vi "Emerson 5700 32 Bit Data.vi"(8 "Error In":errorcluster, 10 "Emerson Flow Meter Data Input":T2={"Mass Flow Rate (Scaled Integer)"=65535, "Density (Scaled Integer)"=8, "Temperature (Scaled Integer)"=69, "Volume Flow Rate (Scaled Integer)"=65535, "Totalizer 1 (Scaled Integer)"=65, "Totalizer 2 (Scaled Integer)"=8, "Transmitter Software Rev"=14, "Flow Direction"="Forward", "Mass Flow Units"="lb/min", "Density Units"="lb/US Gal", "Temperature Units"="°F", "Volume Flow Units"="US GPM", "Pressure Units"="PSI", "Mass Total Units"="lbs", "Volume Total Units"="US Gallon", "Inventory 1 (Scaled Integer)"=66, "Inventory 2 (Scaled Integer)"=8, "Mass Flow Rate"=0.0, "Density"=0.0, "Temperature"=0.0, "Volume Flow Rate"=0.0, "Pressure (Scaled Integer)"=40, "Current Value Totalizer 1 (Pounds per draw)"=0.0, "Current Value Totalizer 2 (Gallons per draw)"=0.0, "Current Value Inventory 1 (Pounds Total)"=0.0, "Current Value Inventory 2 (Gallons Total)"=0.0, "Drive Gain"=0.0, "Raw Tube Frequency (Hz)"=0.0, "Dynamic Viscosity (Centipoise)"=0.0, "Kinematic Viscosity (Centistokes)"=0.0, "Hot Gallons (Calculated Gallons)"=0.0, "Hot Flow Rate (Calculated GPM)"=0.0, "Hot Gallons Inventory (Gallons)"=0.0}, 11 "Modbus master in":refnum<class "Modbus Master.lvclass">=refnum) -> (0 "Error Out":errorcluster, 2 "Emerson Flow Meter Data Output":T2, 3 "Modbus master out":refnum<class "Modbus Master.lvclass">)   [LabVIEW 2016]
uses:
  Type Definitions/Emerson 5700 Data.ctl
  <vilib>/NI/Modbus Library/API/Master/Modbus Master.lvclass
  <vilib>/NI/Modbus Library/Transmission Data Unit/IP/IP Data Unit.lvclass
  <vilib>/NI/Modbus Library/Master Function Definition/Master Function Definition.lvclass
  <vilib>/NI/Modbus Library/Network Protocol/Network Master/TCP/TCP Master.lvclass
  Type Definitions/Emerson 5700 Modbus Addresses.ctl
panel:
  in  "CMD 10":T1=291 items=["Kinematic Viscosity-4161"=4161, "Dynamic Viscosity-4159"=4159, "Reset Volume Total (Totalizer 2)-57"=57, "Reset Mass Total (Totalizer 1)-56"=56, "Drive Gain-291"=291, "Raw Tube Frequency (Hz) - 285"=285, "Current Value Inventory 2-265"=265, "Current Value Inventory 1-263"=263, "Current Value Totalizer 2-261"=261, "Current Value Totalizer 1-259"=259, "Volume Flow Rate-253"=253, "Temperature-251"=251, "Density-249"=249, "Mass Flow Rate-247"=247, "Volume Total Unit-46"=46, "Mass Total Unit-45"=45, "Pressure Unit-44"=44, "Volume Flow Unit-42"=42, "Temperature Unit-41"=41, "Density Unit-40"=40, "Mass Flow Units-39"=39, "Flow Direction-17"=17, "Transmitter Software Rev-16"=16, "Inventory 2 (Scaled Integer)-11"=11, "Inventory 1 (Scaled Integer)-10"=10, "Totalizer 2 (Scaled Integer)-9"=9, "Totalizer 1 (Scaled Integer)-8"=8, "Pressure (Scaled Integer) -7"=7, "Volume Flow Rate (Scaled Integer)-5"=5, "Temperature (Scaled Integer)-4"=4, "Density (Scaled Integer)-3"=3, "Mass Flow Rate (Scaled Integer)-2"=2]
  in  "CMD 9":T1=265 items=["Kinematic Viscosity-4161"=4161, "Dynamic Viscosity-4159"=4159, "Reset Volume Total (Totalizer 2)-57"=57, "Reset Mass Total (Totalizer 1)-56"=56, "Drive Gain-291"=291, "Raw Tube Frequency (Hz) - 285"=285, "Current Value Inventory 2-265"=265, "Current Value Inventory 1-263"=263, "Current Value Totalizer 2-261"=261, "Current Value Totalizer 1-259"=259, "Volume Flow Rate-253"=253, "Temperature-251"=251, "Density-249"=249, "Mass Flow Rate-247"=247, "Volume Total Unit-46"=46, "Mass Total Unit-45"=45, "Pressure Unit-44"=44, "Volume Flow Unit-42"=42, "Temperature Unit-41"=41, "Density Unit-40"=40, "Mass Flow Units-39"=39, "Flow Direction-17"=17, "Transmitter Software Rev-16"=16, "Inventory 2 (Scaled Integer)-11"=11, "Inventory 1 (Scaled Integer)-10"=10, "Totalizer 2 (Scaled Integer)-9"=9, "Totalizer 1 (Scaled Integer)-8"=8, "Pressure (Scaled Integer) -7"=7, "Volume Flow Rate (Scaled Integer)-5"=5, "Temperature (Scaled Integer)-4"=4, "Density (Scaled Integer)-3"=3, "Mass Flow Rate (Scaled Integer)-2"=2]
  in  "CMD 8":T1=263 items=["Kinematic Viscosity-4161"=4161, "Dynamic Viscosity-4159"=4159, "Reset Volume Total (Totalizer 2)-57"=57, "Reset Mass Total (Totalizer 1)-56"=56, "Drive Gain-291"=291, "Raw Tube Frequency (Hz) - 285"=285, "Current Value Inventory 2-265"=265, "Current Value Inventory 1-263"=263, "Current Value Totalizer 2-261"=261, "Current Value Totalizer 1-259"=259, "Volume Flow Rate-253"=253, "Temperature-251"=251, "Density-249"=249, "Mass Flow Rate-247"=247, "Volume Total Unit-46"=46, "Mass Total Unit-45"=45, "Pressure Unit-44"=44, "Volume Flow Unit-42"=42, "Temperature Unit-41"=41, "Density Unit-40"=40, "Mass Flow Units-39"=39, "Flow Direction-17"=17, "Transmitter Software Rev-16"=16, "Inventory 2 (Scaled Integer)-11"=11, "Inventory 1 (Scaled Integer)-10"=10, "Totalizer 2 (Scaled Integer)-9"=9, "Totalizer 1 (Scaled Integer)-8"=8, "Pressure (Scaled Integer) -7"=7, "Volume Flow Rate (Scaled Integer)-5"=5, "Temperature (Scaled Integer)-4"=4, "Density (Scaled Integer)-3"=3, "Mass Flow Rate (Scaled Integer)-2"=2]
  in  "CMD 7":T1=261 items=["Kinematic Viscosity-4161"=4161, "Dynamic Viscosity-4159"=4159, "Reset Volume Total (Totalizer 2)-57"=57, "Reset Mass Total (Totalizer 1)-56"=56, "Drive Gain-291"=291, "Raw Tube Frequency (Hz) - 285"=285, "Current Value Inventory 2-265"=265, "Current Value Inventory 1-263"=263, "Current Value Totalizer 2-261"=261, "Current Value Totalizer 1-259"=259, "Volume Flow Rate-253"=253, "Temperature-251"=251, "Density-249"=249, "Mass Flow Rate-247"=247, "Volume Total Unit-46"=46, "Mass Total Unit-45"=45, "Pressure Unit-44"=44, "Volume Flow Unit-42"=42, "Temperature Unit-41"=41, "Density Unit-40"=40, "Mass Flow Units-39"=39, "Flow Direction-17"=17, "Transmitter Software Rev-16"=16, "Inventory 2 (Scaled Integer)-11"=11, "Inventory 1 (Scaled Integer)-10"=10, "Totalizer 2 (Scaled Integer)-9"=9, "Totalizer 1 (Scaled Integer)-8"=8, "Pressure (Scaled Integer) -7"=7, "Volume Flow Rate (Scaled Integer)-5"=5, "Temperature (Scaled Integer)-4"=4, "Density (Scaled Integer)-3"=3, "Mass Flow Rate (Scaled Integer)-2"=2]
  in  "CMD 6":T1=259 items=["Kinematic Viscosity-4161"=4161, "Dynamic Viscosity-4159"=4159, "Reset Volume Total (Totalizer 2)-57"=57, "Reset Mass Total (Totalizer 1)-56"=56, "Drive Gain-291"=291, "Raw Tube Frequency (Hz) - 285"=285, "Current Value Inventory 2-265"=265, "Current Value Inventory 1-263"=263, "Current Value Totalizer 2-261"=261, "Current Value Totalizer 1-259"=259, "Volume Flow Rate-253"=253, "Temperature-251"=251, "Density-249"=249, "Mass Flow Rate-247"=247, "Volume Total Unit-46"=46, "Mass Total Unit-45"=45, "Pressure Unit-44"=44, "Volume Flow Unit-42"=42, "Temperature Unit-41"=41, "Density Unit-40"=40, "Mass Flow Units-39"=39, "Flow Direction-17"=17, "Transmitter Software Rev-16"=16, "Inventory 2 (Scaled Integer)-11"=11, "Inventory 1 (Scaled Integer)-10"=10, "Totalizer 2 (Scaled Integer)-9"=9, "Totalizer 1 (Scaled Integer)-8"=8, "Pressure (Scaled Integer) -7"=7, "Volume Flow Rate (Scaled Integer)-5"=5, "Temperature (Scaled Integer)-4"=4, "Density (Scaled Integer)-3"=3, "Mass Flow Rate (Scaled Integer)-2"=2]
  in  "CMD 5":T1=285 items=["Kinematic Viscosity-4161"=4161, "Dynamic Viscosity-4159"=4159, "Reset Volume Total (Totalizer 2)-57"=57, "Reset Mass Total (Totalizer 1)-56"=56, "Drive Gain-291"=291, "Raw Tube Frequency (Hz) - 285"=285, "Current Value Inventory 2-265"=265, "Current Value Inventory 1-263"=263, "Current Value Totalizer 2-261"=261, "Current Value Totalizer 1-259"=259, "Volume Flow Rate-253"=253, "Temperature-251"=251, "Density-249"=249, "Mass Flow Rate-247"=247, "Volume Total Unit-46"=46, "Mass Total Unit-45"=45, "Pressure Unit-44"=44, "Volume Flow Unit-42"=42, "Temperature Unit-41"=41, "Density Unit-40"=40, "Mass Flow Units-39"=39, "Flow Direction-17"=17, "Transmitter Software Rev-16"=16, "Inventory 2 (Scaled Integer)-11"=11, "Inventory 1 (Scaled Integer)-10"=10, "Totalizer 2 (Scaled Integer)-9"=9, "Totalizer 1 (Scaled Integer)-8"=8, "Pressure (Scaled Integer) -7"=7, "Volume Flow Rate (Scaled Integer)-5"=5, "Temperature (Scaled Integer)-4"=4, "Density (Scaled Integer)-3"=3, "Mass Flow Rate (Scaled Integer)-2"=2]
  in  "CMD 4":T1=253 items=["Kinematic Viscosity-4161"=4161, "Dynamic Viscosity-4159"=4159, "Reset Volume Total (Totalizer 2)-57"=57, "Reset Mass Total (Totalizer 1)-56"=56, "Drive Gain-291"=291, "Raw Tube Frequency (Hz) - 285"=285, "Current Value Inventory 2-265"=265, "Current Value Inventory 1-263"=263, "Current Value Totalizer 2-261"=261, "Current Value Totalizer 1-259"=259, "Volume Flow Rate-253"=253, "Temperature-251"=251, "Density-249"=249, "Mass Flow Rate-247"=247, "Volume Total Unit-46"=46, "Mass Total Unit-45"=45, "Pressure Unit-44"=44, "Volume Flow Unit-42"=42, "Temperature Unit-41"=41, "Density Unit-40"=40, "Mass Flow Units-39"=39, "Flow Direction-17"=17, "Transmitter Software Rev-16"=16, "Inventory 2 (Scaled Integer)-11"=11, "Inventory 1 (Scaled Integer)-10"=10, "Totalizer 2 (Scaled Integer)-9"=9, "Totalizer 1 (Scaled Integer)-8"=8, "Pressure (Scaled Integer) -7"=7, "Volume Flow Rate (Scaled Integer)-5"=5, "Temperature (Scaled Integer)-4"=4, "Density (Scaled Integer)-3"=3, "Mass Flow Rate (Scaled Integer)-2"=2]
  in  "CMD 3":T1=251 items=["Kinematic Viscosity-4161"=4161, "Dynamic Viscosity-4159"=4159, "Reset Volume Total (Totalizer 2)-57"=57, "Reset Mass Total (Totalizer 1)-56"=56, "Drive Gain-291"=291, "Raw Tube Frequency (Hz) - 285"=285, "Current Value Inventory 2-265"=265, "Current Value Inventory 1-263"=263, "Current Value Totalizer 2-261"=261, "Current Value Totalizer 1-259"=259, "Volume Flow Rate-253"=253, "Temperature-251"=251, "Density-249"=249, "Mass Flow Rate-247"=247, "Volume Total Unit-46"=46, "Mass Total Unit-45"=45, "Pressure Unit-44"=44, "Volume Flow Unit-42"=42, "Temperature Unit-41"=41, "Density Unit-40"=40, "Mass Flow Units-39"=39, "Flow Direction-17"=17, "Transmitter Software Rev-16"=16, "Inventory 2 (Scaled Integer)-11"=11, "Inventory 1 (Scaled Integer)-10"=10, "Totalizer 2 (Scaled Integer)-9"=9, "Totalizer 1 (Scaled Integer)-8"=8, "Pressure (Scaled Integer) -7"=7, "Volume Flow Rate (Scaled Integer)-5"=5, "Temperature (Scaled Integer)-4"=4, "Density (Scaled Integer)-3"=3, "Mass Flow Rate (Scaled Integer)-2"=2]
  in  "CMD 2":T1=249 items=["Kinematic Viscosity-4161"=4161, "Dynamic Viscosity-4159"=4159, "Reset Volume Total (Totalizer 2)-57"=57, "Reset Mass Total (Totalizer 1)-56"=56, "Drive Gain-291"=291, "Raw Tube Frequency (Hz) - 285"=285, "Current Value Inventory 2-265"=265, "Current Value Inventory 1-263"=263, "Current Value Totalizer 2-261"=261, "Current Value Totalizer 1-259"=259, "Volume Flow Rate-253"=253, "Temperature-251"=251, "Density-249"=249, "Mass Flow Rate-247"=247, "Volume Total Unit-46"=46, "Mass Total Unit-45"=45, "Pressure Unit-44"=44, "Volume Flow Unit-42"=42, "Temperature Unit-41"=41, "Density Unit-40"=40, "Mass Flow Units-39"=39, "Flow Direction-17"=17, "Transmitter Software Rev-16"=16, "Inventory 2 (Scaled Integer)-11"=11, "Inventory 1 (Scaled Integer)-10"=10, "Totalizer 2 (Scaled Integer)-9"=9, "Totalizer 1 (Scaled Integer)-8"=8, "Pressure (Scaled Integer) -7"=7, "Volume Flow Rate (Scaled Integer)-5"=5, "Temperature (Scaled Integer)-4"=4, "Density (Scaled Integer)-3"=3, "Mass Flow Rate (Scaled Integer)-2"=2]
  in  "CMD 1":T1=247 items=["Kinematic Viscosity-4161"=4161, "Dynamic Viscosity-4159"=4159, "Reset Volume Total (Totalizer 2)-57"=57, "Reset Mass Total (Totalizer 1)-56"=56, "Drive Gain-291"=291, "Raw Tube Frequency (Hz) - 285"=285, "Current Value Inventory 2-265"=265, "Current Value Inventory 1-263"=263, "Current Value Totalizer 2-261"=261, "Current Value Totalizer 1-259"=259, "Volume Flow Rate-253"=253, "Temperature-251"=251, "Density-249"=249, "Mass Flow Rate-247"=247, "Volume Total Unit-46"=46, "Mass Total Unit-45"=45, "Pressure Unit-44"=44, "Volume Flow Unit-42"=42, "Temperature Unit-41"=41, "Density Unit-40"=40, "Mass Flow Units-39"=39, "Flow Direction-17"=17, "Transmitter Software Rev-16"=16, "Inventory 2 (Scaled Integer)-11"=11, "Inventory 1 (Scaled Integer)-10"=10, "Totalizer 2 (Scaled Integer)-9"=9, "Totalizer 1 (Scaled Integer)-8"=8, "Pressure (Scaled Integer) -7"=7, "Volume Flow Rate (Scaled Integer)-5"=5, "Temperature (Scaled Integer)-4"=4, "Density (Scaled Integer)-3"=3, "Mass Flow Rate (Scaled Integer)-2"=2]
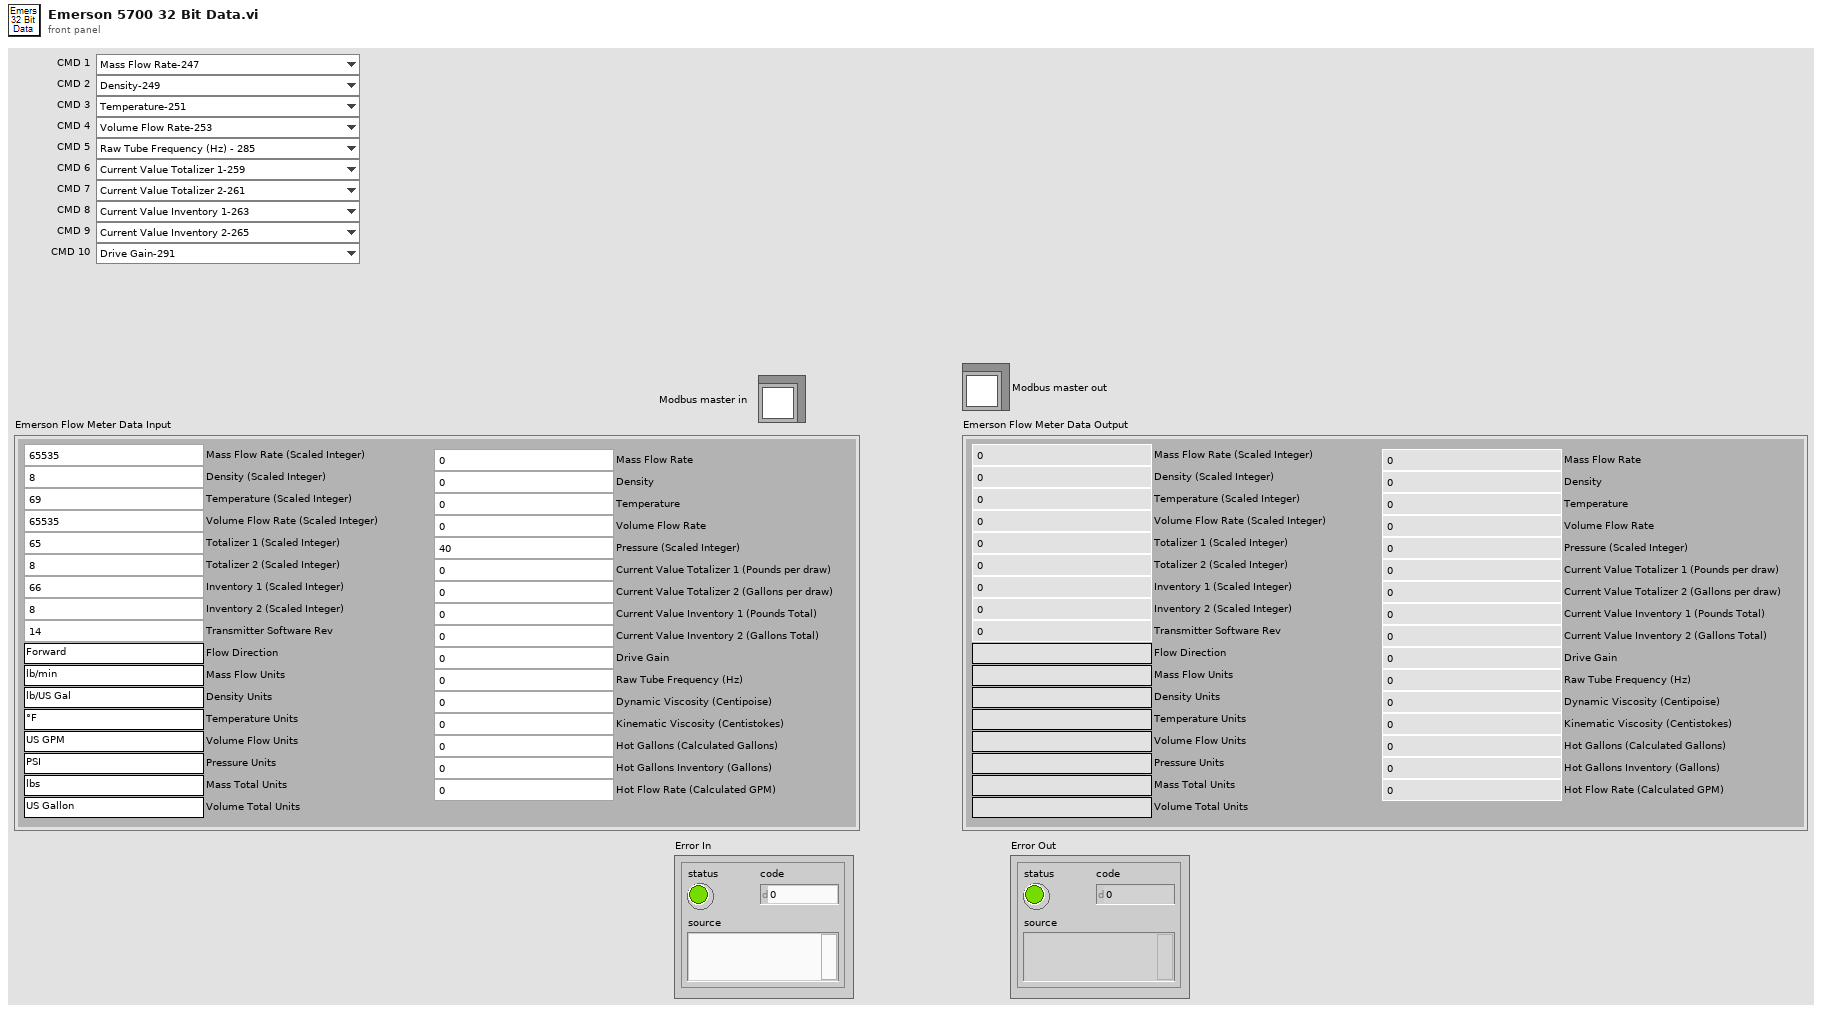
[diagram p1: front panel]
types:
  T1 = typedef "Emerson 5700 Modbus Addresses.ctl" = u16
  T2 = typedef "Emerson 5700 Data.ctl" = cluster{"Mass Flow Rate (Scaled Integer)":u16, "Density (Scaled Integer)":u16, "Temperature (Scaled Integer)":u16, "Volume Flow Rate (Scaled Integer)":u16, "Totalizer 1 (Scaled Integer)":u16, "Totalizer 2 (Scaled Integer)":u16, "Transmitter Software Rev":u16, "Flow Direction":string, "Mass Flow Units":string, "Density Units":string, "Temperature Units":string, "Volume Flow Units":string, "Pressure Units":string, "Mass Total Units":string, "Volume Total Units":string, "Inventory 1 (Scaled Integer)":u16, "Inventory 2 (Scaled Integer)":u16, "Mass Flow Rate":dbl, "Density":dbl, "Temperature":dbl, "Volume Flow Rate":dbl, "Pressure (Scaled Integer)":u16, "Current Value Totalizer 1 (Pounds per draw)":dbl, "Current Value Totalizer 2 (Gallons per draw)":dbl, "Current Value Inventory 1 (Pounds Total)":dbl, "Current Value Inventory 2 (Gallons Total)":dbl, "Drive Gain":dbl, "Raw Tube Frequency (Hz)":dbl, "Dynamic Viscosity (Centipoise)":dbl, "Kinematic Viscosity (Centistokes)":dbl, "Hot Gallons (Calculated Gallons)":dbl, "Hot Flow Rate (Calculated GPM)":dbl, "Hot Gallons Inventory (Gallons)":dbl}
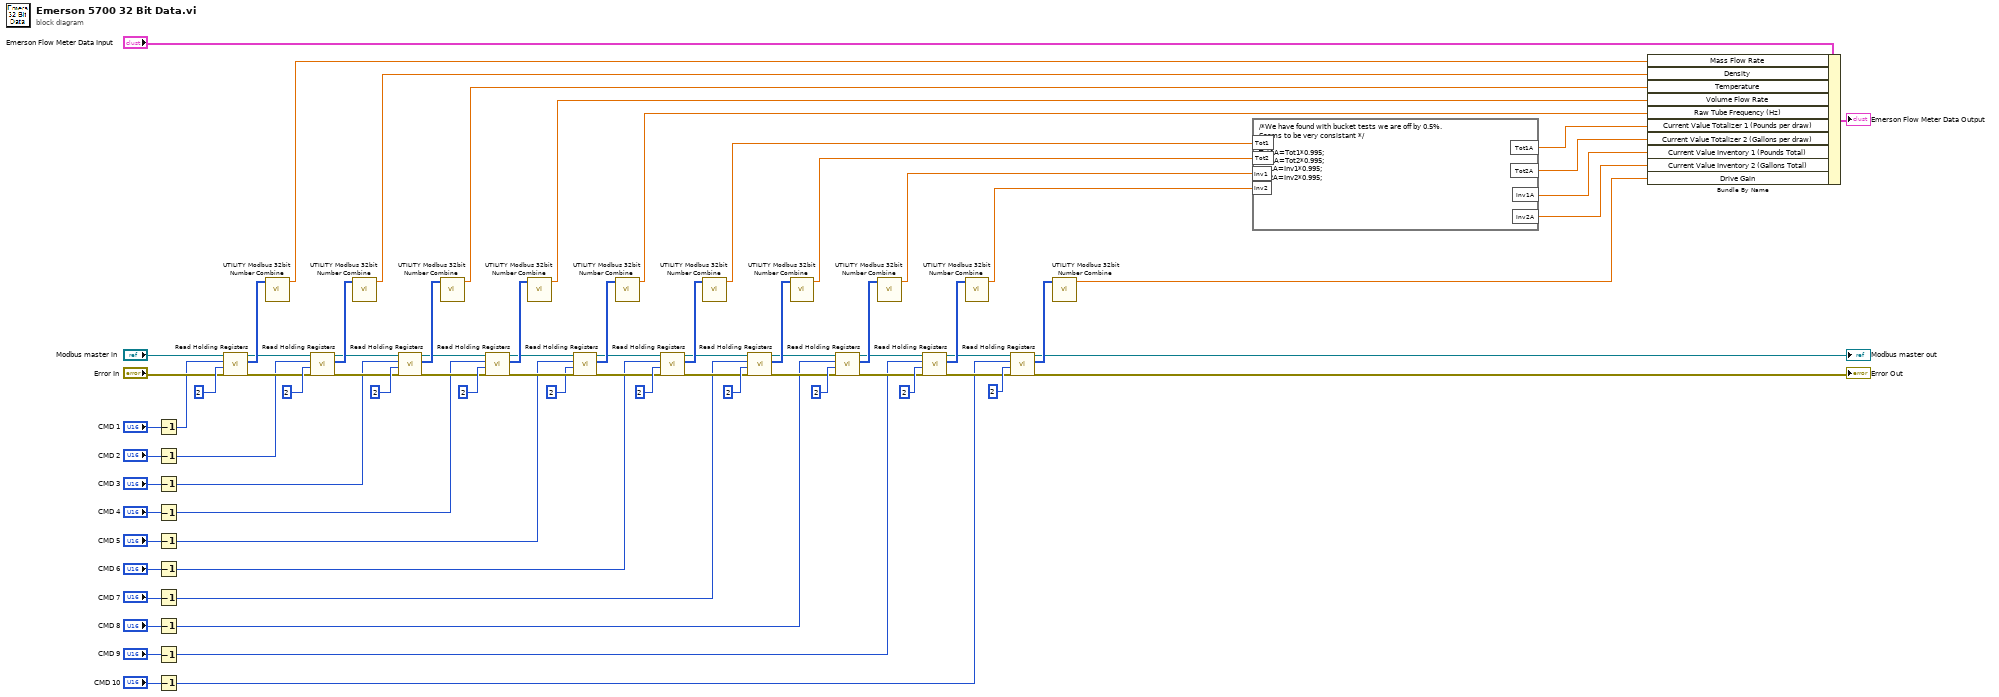
[diagram p0: block diagram]
diagram:
  n1 = Decrement(x="CMD 1") -> (x-1=w30:T1)
  n2 = Decrement(x="CMD 2") -> (x-1=w28:T1)
  n3 = Decrement(x="CMD 3") -> (x-1=w26:T1)
  n4 = Decrement(x="CMD 4") -> (x-1=w24:T1)
  n5 = Decrement(x="CMD 5") -> (x-1=w22:T1)
  n6 = Decrement(x="CMD 6") -> (x-1=w20:T1)
  n7 = Decrement(x="CMD 7") -> (x-1=w18:T1)
  n8 = Decrement(x="CMD 8") -> (x-1=w16:T1)
  n9 = Decrement(x="CMD 9") -> (x-1=w14:T1)
  n10 = Decrement(x="CMD 10") -> (x-1=w12:T1)
  n11 = call-dynamic "Read Holding Registers.vi"("error in"="Error In", "number of inputs"=u16 2 ("Quantity"), "starting address"=w30, "Modbus master in"="Modbus master in") -> ("error out"=w63:errorcluster, "register values"=w77:u16[], "Modbus master out"=w67:refnum<class "Modbus Master.lvclass">)  [unwired: 5 in]
  n12 = call "UTILITY Modbus 32bit Number Combine.vi"("Holding Registers"=w77) -> ("Data"=w38:sgl)  [unwired: 9 in, 1 out]
  n13 = call-dynamic "Read Holding Registers.vi"("error in"=w63, "number of inputs"=u16 2 ("Quantity"), "starting address"=w28, "Modbus master in"=w67) -> ("error out"=w62:errorcluster, "register values"=w74:u16[], "Modbus master out"=w66:refnum<class "Modbus Master.lvclass">)  [unwired: 5 in]
  n14 = call "UTILITY Modbus 32bit Number Combine.vi"("Holding Registers"=w74) -> ("Data"=w37:sgl)  [unwired: 9 in, 1 out]
  n15 = call-dynamic "Read Holding Registers.vi"("error in"=w62, "number of inputs"=u16 2 ("Quantity"), "starting address"=w26, "Modbus master in"=w66) -> ("error out"=w61:errorcluster, "register values"=w71:u16[], "Modbus master out"=w65:refnum<class "Modbus Master.lvclass">)  [unwired: 5 in]
  n16 = call "UTILITY Modbus 32bit Number Combine.vi"("Holding Registers"=w71) -> ("Data"=w36:sgl)  [unwired: 9 in, 1 out]
  n17 = call-dynamic "Read Holding Registers.vi"("error in"=w61, "number of inputs"=u16 2 ("Quantity"), "starting address"=w24, "Modbus master in"=w65) -> ("error out"=w60:errorcluster, "register values"=w70:u16[], "Modbus master out"=w64:refnum<class "Modbus Master.lvclass">)  [unwired: 5 in]
  n18 = call "UTILITY Modbus 32bit Number Combine.vi"("Holding Registers"=w70) -> ("Data"=w35:sgl)  [unwired: 9 in, 1 out]
  n19 = call-dynamic "Read Holding Registers.vi"("error in"=w60, "number of inputs"=u16 2 ("Quantity"), "starting address"=w22, "Modbus master in"=w64) -> ("error out"=w49:errorcluster, "register values"=w68:u16[], "Modbus master out"=w44:refnum<class "Modbus Master.lvclass">)  [unwired: 5 in]
  n20 = call "UTILITY Modbus 32bit Number Combine.vi"("Holding Registers"=w68) -> ("Data"=w34:sgl)  [unwired: 9 in, 1 out]
  n21 = call-dynamic "Read Holding Registers.vi"("error in"=w49, "number of inputs"=u16 2 ("Quantity"), "starting address"=w20, "Modbus master in"=w44) -> ("error out"=w48:errorcluster, "register values"=w59:u16[], "Modbus master out"=w43:refnum<class "Modbus Master.lvclass">)  [unwired: 5 in]
  n22 = call "UTILITY Modbus 32bit Number Combine.vi"("Holding Registers"=w59) -> ("Data"=w8:sgl)  [unwired: 9 in, 1 out]
  n23 = call-dynamic "Read Holding Registers.vi"("error in"=w48, "number of inputs"=u16 2 ("Quantity"), "starting address"=w18, "Modbus master in"=w43) -> ("error out"=w47:errorcluster, "register values"=w56:u16[], "Modbus master out"=w42:refnum<class "Modbus Master.lvclass">)  [unwired: 5 in]
  n24 = call "UTILITY Modbus 32bit Number Combine.vi"("Holding Registers"=w56) -> ("Data"=w7:sgl)  [unwired: 9 in, 1 out]
  n25 = call-dynamic "Read Holding Registers.vi"("error in"=w47, "number of inputs"=u16 2 ("Quantity"), "starting address"=w16, "Modbus master in"=w42) -> ("error out"=w46:errorcluster, "register values"=w55:u16[], "Modbus master out"=w41:refnum<class "Modbus Master.lvclass">)  [unwired: 5 in]
  n26 = call "UTILITY Modbus 32bit Number Combine.vi"("Holding Registers"=w55) -> ("Data"=w6:sgl)  [unwired: 9 in, 1 out]
  n27 = call-dynamic "Read Holding Registers.vi"("error in"=w46, "number of inputs"=u16 2 ("Quantity"), "starting address"=w14, "Modbus master in"=w41) -> ("error out"=w45:errorcluster, "register values"=w52:u16[], "Modbus master out"=w40:refnum<class "Modbus Master.lvclass">)  [unwired: 5 in]
  n28 = call "UTILITY Modbus 32bit Number Combine.vi"("Holding Registers"=w52) -> ("Data"=w5:sgl)  [unwired: 9 in, 1 out]
  n29 = call-dynamic "Read Holding Registers.vi"("error in"=w45, "number of inputs"=u16 2 ("Quantity"), "starting address"=w12, "Modbus master in"=w40) -> ("error out"=→"Error Out":errorcluster, "register values"=w51:u16[], "Modbus master out"=→"Modbus master out":refnum<class "Modbus Master.lvclass">)  [unwired: 5 in]
  n30 = call "UTILITY Modbus 32bit Number Combine.vi"("Holding Registers"=w51) -> ("Data"=w33:sgl)  [unwired: 9 in, 1 out]
  n31 = formula code="/*We have found with bucket tests we are off by 0.5%.\nSeems to be very consistant */\n\nTot1A=Tot1*0.995;\nTot2A=Tot2*0.995;\nInv1A=Inv1*0.995;\nInv2A=Inv2*0.995;"("Tot1"=w8, "Tot2"=w7, "Inv1"=w6, "Inv2"=w5) -> ("Tot1A"=w4:dbl, "Tot2A"=w3:dbl, "Inv1A"=w2:dbl, "Inv2A"=w1:dbl)
  n32 = Bundle By Name(cluster="Emerson Flow Meter Data Input", "Mass Flow Rate"=w38, "Density"=w37, "Temperature"=w36, "Volume Flow Rate"=w35, "Raw Tube Frequency (Hz)"=w34, "Current Value Totalizer 1 (Pounds per draw)"=w4, "Current Value Totalizer 2 (Gallons per draw)"=w3, "Current Value Inventory 1 (Pounds Total)"=w2, "Current Value Inventory 2 (Gallons Total)"=w1, "Drive Gain"=w33) -> (→"Emerson Flow Meter Data Output":T2)
